vi "Recursive list files.vi"(8 "error in (no error)":errorcluster, 11 "Folders":path[](array[path])) -> (0 "error out":errorcluster, 2 "All Files in Hierarchy":path[](array[path]))   [LabVIEW 2020, in "Method Generation.lvlib" / "Getter Generator.lvclass"]
uses:
  Getter Generator.lvclass
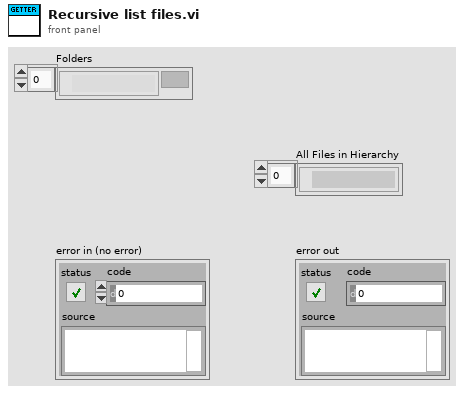
[diagram p1: front panel]
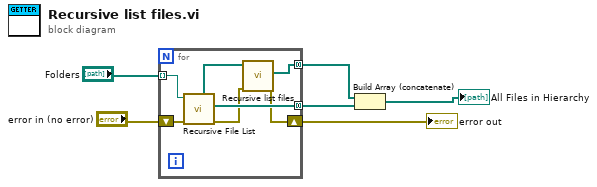
[diagram p0: block diagram]
diagram:
  n1 = for {
    tunnel: "Folders" -> [w11] mode=indexing
    tunnel: [w13] -> w4 mode=concatenating
    shift-right: [w8] -> w6
    shift-left: "error in (no error)" -> [w12]
    tunnel: [w7] -> w2 mode=concatenating
    n2 = call <vilib>:"Recursive File List.vi"("error in (no error)"=w12, "Folder Path"=w11) -> ("error out"=w9:errorcluster, "All Files in Dir"=w13:path[], "All Folders"=w10:path[])  [unwired: 5 in, 2 out]
    n3 = call "Recursive list files.vi"("error in (no error)"=w9, "Folders"=w10) -> ("error out"=w8:errorcluster, "All Files in Hierarchy"=w7:path[])  [unwired: 8 in]
  }
  "error out" <- w6
  n4 = Build Array (concatenate)(w2, w4) -> (→"All Files in Hierarchy":path[])
